vi "Chroma 19052 Set Test Params.vi"() -> ()   [LabVIEW 2025]
uses:
  Support/AC parameters--cluster.ctl
  Support/DC parameters--cluster.ctl
  Support/IR parameters--cluster.ctl
  <instrlib>/Chroma 19052/Public/Utility/Type Def/steps--numeric.ctl
  <instrlib>/Chroma 19052/Chroma 19052.lvlib
panel:
  out "Instrument Info":string[](array[string])
  in  "IR Parameters":T1={"Voltage Level [V]"=500, "Hi Limit [ohm]"=30000000000.0, "Test Time [s] "=1.3, "Dwell Time [s]"=4.4, "Lo Limit [ohm]"=2500000.0, "Ramp Time [s] "=1.1, "Fall Time [s]"=2.2} {"Voltage Level [V]" min=50 max=1000 step=1 format="%.3p"; "Hi Limit [ohm]" min=0.0 max=50000000000000.0 step=100000.0 format="%.1p"; "Test Time [s]" min=0.0 max=999.0 step=0.1 format="%.1p"; "Dwell Time [s]" min=0.0 max=999.0 step=0.1 format="%.1p"; "Lo Limit [ohm]" min=100000.0 max=50000000000000.0 step=100000.0 format="%.1p"; "Ramp Time [s]" min=0.0 max=999.0 step=0.1 format="%.1p"; "Fall Time [s]" min=0.0 max=999.0 step=0.1 format="%.1p"}
  in  "DC Parameters":T2={"Voltage Level [V]"=1000, "Hi Limit [A]"=0.005, "Test Time [s] "=2.3, "Dwell Time [s]"=4.4, "Lo Limit [A]"=0.0, "ARC Limit [A]"=0.005, "Ramp Time [s] "=1.1, "Fall Time [s]"=2.2} {"Voltage Level [V]" min=50 max=6000 step=1 format="%.3p"; "Hi Limit [A]" min=1e-07 max=0.01 step=1e-07 format="%.2p"; "Test Time [s]" min=0.0 max=999.0 step=0.1 format="%.1p"; "Dwell Time [s]" min=0.0 max=999.0 step=0.1 format="%.1p"; "Lo Limit [A]" min=0.0 max=0.01 step=1e-06 format="%.2p"; "ARC Limit [A]" min=0.0 max=0.01 step=0.001 format="%.1p"; "Ramp Time [s]" min=0.0 max=999.0 step=0.1 format="%.1p"; "Fall Time [s]" min=0.0 max=999.0 step=0.1 format="%.1p"}
  in  "AC Parameters":T3={"Voltage Level [V] "=1500, "Hi Limit [A]"=0.01, "Test Time [s] "=3.3, "Lo Limit [A]"=1e-05, "ARC Limit [A]"=0.007, "Ramp Time [s] "=1.1, "Fall Time [s]"=2.2} {"Voltage Level [V]" min=50 max=5000 step=1 format="%.3p"; "Hi Limit [A]" min=0.0001 max=0.03 step=1e-07 format="%.2p"; "Test Time [s]" min=0.0 max=999.0 step=0.1 format="%.1p"; "Lo Limit [A]" min=0.0 max=0.03 step=1e-07 format="%.2p"; "ARC Limit [A]" min=0.0 max=15.0 format="%.1p"; "Ramp Time [s]" min=0.0 max=999.0 step=0.1 format="%.1p"; "Fall Time [s]" min=0.0 max=999.0 step=0.1 format="%.1p"}
  in  "Serial Configuration":T4={"Baud Rate"=9600, "Flow Control"=0, "Parity"=0, "Data Bits"=8} {"Baud Rate" items=["300"=300, "600"=600, "1200"=1200, "2400"=2400, "4800"=4800, "9600"=9600, "19200"=19200]; "Flow Control" items=["NONE", "SOFTWARE"]; "Parity" items=["NONE", "ODD", "EVEN"]; "Data Bits" items=["7"=7, "8"=8]}
  in  "VISA resource name":refnum<visa-resource-name>="Hi-Pot_COM6"
  # "Step 1 AC"
  # "Step 2 DC"
  # "Step 3 IR"
  # "19052 SET TEST \nPARAMETERS"
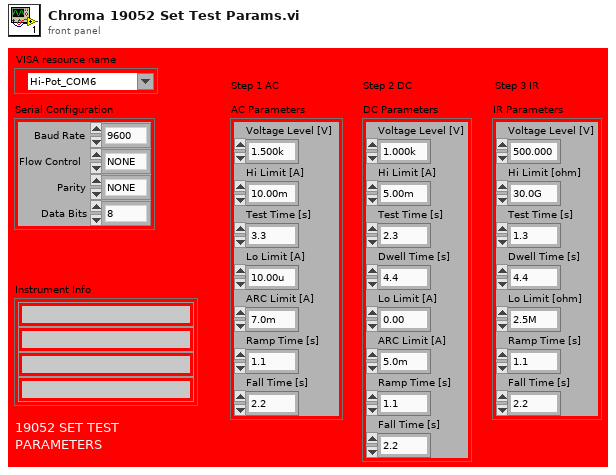
[diagram p1: front panel]
types:
  T1 = typedef "IR parameters--cluster.ctl" = cluster{"Voltage Level [V]":u16, "Hi Limit [ohm]":dbl, "Test Time [s] ":dbl, "Dwell Time [s]":dbl, "Lo Limit [ohm]":dbl, "Ramp Time [s] ":dbl, "Fall Time [s]":dbl}
  T2 = typedef "DC parameters--cluster.ctl" = cluster{"Voltage Level [V]":u16, "Hi Limit [A]":dbl, "Test Time [s] ":dbl, "Dwell Time [s]":dbl, "Lo Limit [A]":dbl, "ARC Limit [A]":dbl, "Ramp Time [s] ":dbl, "Fall Time [s]":dbl}
  T3 = typedef "AC parameters--cluster.ctl" = cluster{"Voltage Level [V] ":u16, "Hi Limit [A]":dbl, "Test Time [s] ":dbl, "Lo Limit [A]":dbl, "ARC Limit [A]":dbl, "Ramp Time [s] ":dbl, "Fall Time [s]":dbl}
  T4 = cluster{"Baud Rate":u32, "Flow Control":u16, "Parity":u16, "Data Bits":u16}
  T5 = typedef "Chroma 19052.lvlib/steps--numeric.ctl" = u8
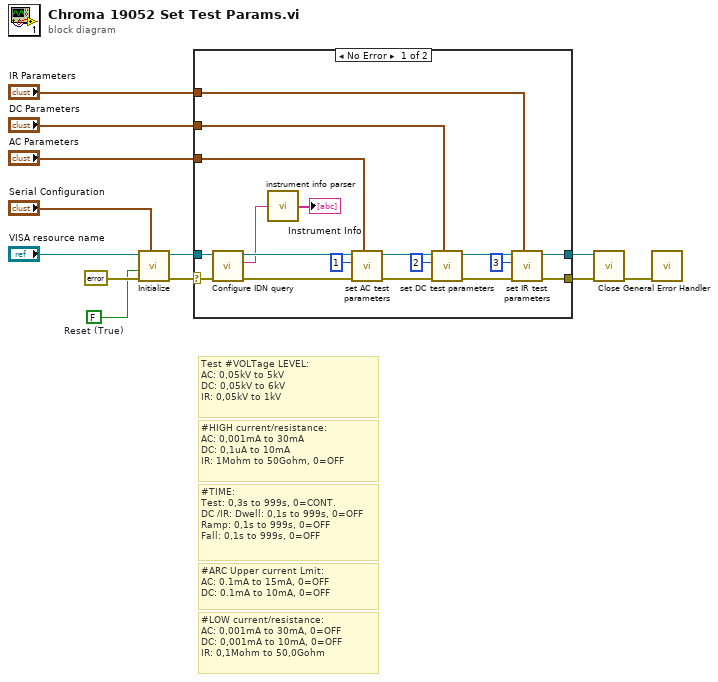
[diagram p0: block diagram]
diagram:
  w1 = FALSE  # Reset (True)
  # "#ARC Upper current Lmit:\nAC: 0.1mA to 15mA, 0=OFF\nDC: 0.1mA to 10mA, 0=OFF"
  # "#TIME: \nTest: 0,3s to 999s, 0=CONT. \nDC /IR: Dwell: 0,1s to 999s, 0=OFF\nRamp: 0,1s to 999s, 0=OFF\nFall: 0,1s to 999s, 0=OFF"
  # "#LOW current/resistance: \nAC: 0,001mA to 30mA, 0=OFF\nDC: 0,001mA to 10mA, 0=OFF\nIR: 0,1Mohm to 50,0Gohm"
  # "#HIGH current/resistance: \nAC: 0,001mA to 30mA\nDC: 0,1uA to 10mA\nIR: 1Mohm to 50Gohm, 0=OFF"
  # "Test #VOLTage LEVEL: \nAC: 0,05kV to 5kV\nDC: 0,05kV to 6kV\nIR: 0,05kV to 1kV"
  n1 = call <instrlib>:"Initialize.vi"("Serial Configuration"="Serial Configuration", "error in (no error)"=errorcluster {"status"=FALSE, "code"=0, "source"=""}, "Reset (True)"=w1, "VISA resource name"="VISA resource name") -> ("error out"=w2:errorcluster, "VISA resource name out"=w8:refnum<visa-resource-name>)  [unwired: 6 in]
  n2 = case shown="No Error" w2 {
    selector: w2 -> [w21 w32]
    tunnel: w8 -> [w20 w31]
    tunnel: [w26 w32] -> w7
    tunnel: [w25 w31] -> w6
    tunnel: "AC Parameters" -> [w24 _]
    tunnel: "DC Parameters" -> [w23 _]
    tunnel: "IR Parameters" -> [w22 _]
    frame No Error {
      n3 = call <instrlib>:"Configure IDN query.vi"("error in (no error)"=w21, "VISA resource name"=w20) -> ("error out"=w18:errorcluster, "Result"=w17:string, "VISA resource name out"=w19:refnum<visa-resource-name>)  [unwired: 7 in]
      n4 = call "instrument info parser.vi"("ID"=w17) -> ("Instrument Info"=→"Instrument Info":string[])  [unwired: 4 in]
      n5 = call "set AC test parameters.vi"("AC Parameters"=w24, "error in (no error)"=w18, "Step"=T5 1, "VISA Refnum in"=w19) -> ("error out"=w30:errorcluster, "VISA Refnum out"=w29:refnum<visa-resource-name>)  [unwired: 6 in]
      n6 = call "set DC test parameters.vi"("DC Parameters"=w23, "error in (no error)"=w30, "Step"=T5 2, "VISA Refnum in"=w29) -> ("error out"=w27:errorcluster, "VISA Refnum out"=w28:refnum<visa-resource-name>)  [unwired: 6 in]
      n7 = call "set IR test parameters.vi"("IR Parameters"=w22, "error in (no error)"=w27, "Step"=T5 3, "VISA Refnum in"=w28) -> ("error out"=w26:errorcluster, "VISA Refnum out"=w25:refnum<visa-resource-name>)  [unwired: 6 in]
    }
    frame Error {
    }
  }
  n8 = call <instrlib>:"Close.vi"("error in (no error)"=w7, "VISA resource name"=w6) -> ("error out"=w9:errorcluster)  [unwired: 9 in]
  n9 = call <vilib>:"General Error Handler.vi"("error in (no error)"=w9) -> ()  [unwired: 10 in, 5 out]
